vi "Event Contract User.vi"(8 "error in (no error)":errorcluster, 11 "[V] Login in":refnum<class "[V] Login.lvclass">) -> (0 "error out":errorcluster, 3 "[V] Login out":refnum<class "[V] Login.lvclass">)   [LabVIEW 2020, in "[V] Login.lvlib" / "[V] Login.lvclass"]
uses:
  [V] Login.lvclass
  [V] Login.lvclass/[V] Login.ctl
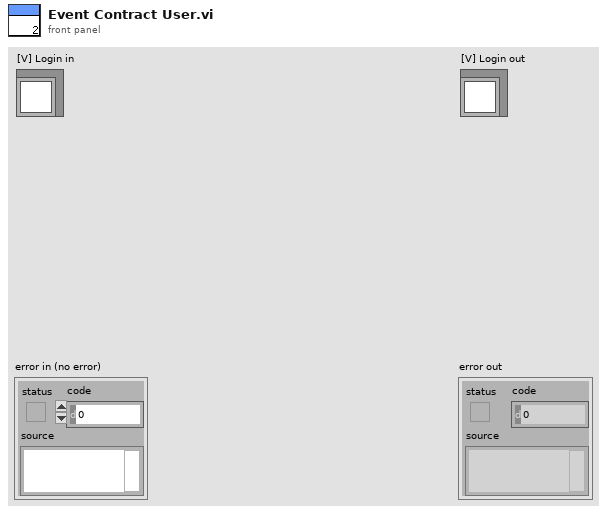
[diagram p1: front panel]
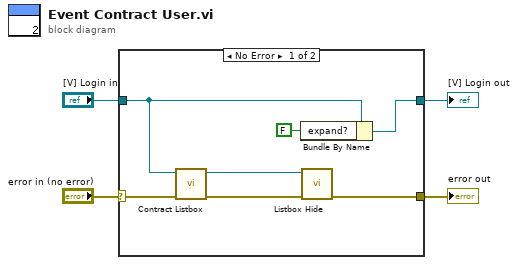
[diagram p0: block diagram]
diagram:
  n1 = case shown="No Error" "error in (no error)" {
    selector: "error in (no error)" -> [w9 w13]
    tunnel: [w5 w13] -> w3
    tunnel: [w11 w12] -> w1
    tunnel: "[V] Login in" -> [w8 w12]
    frame No Error {
      n2 = call "Contract Listbox.vi"("error in (no error)"=w9, "[V] Login in"=w8) -> ("error out"=w7:errorcluster, "[V] Login out"=w6:refnum<class "[V] Login.lvclass">)  [unwired: 8 in]
      n3 = Bundle By Name(cluster=w8, "expand?"=FALSE) -> (w11:refnum<class "[V] Login.lvclass">)
      n4 = call "Listbox Hide.vi"("error in (no error)"=w7, "[V] Login in"=w6) -> ("error out"=w5:errorcluster)  [unwired: 8 in, 1 out]
    }
    frame Error {
    }
  }
  "error out" <- w3
  "[V] Login out" <- w1
